vi "Zaber A Series Move.vi"() -> ()   [LabVIEW 2013]
doc: "This beginner example shows the Move VI, which allows the user to move devices based on real-world units easily."
uses:
  <instrlib>/Zaber A Series/Zaber A Series.lvlib
panel:
  in  "Units (0: microsteps)":u16(ring) items=["microsteps", "microns", "millimeters", "inches"]
  in  "Movement Type (0: relative)":u16(ring) items=["relative", "absolute"]
  in  "Device and Axis":string="1"
  in  "Microstep Size (0)":dbl=0.124023
  in  "Move Distance (0)":dbl
  in  "VISA resource name":refnum<visa-resource-name>="COM5"
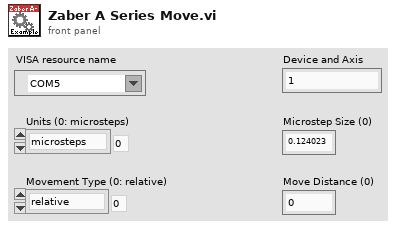
[diagram p1: front panel]
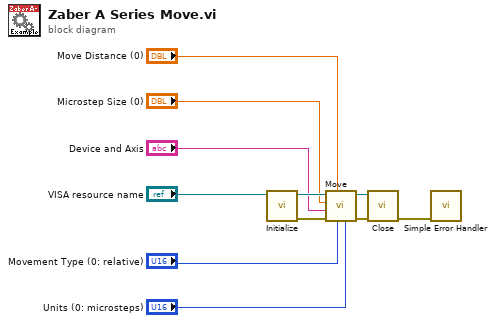
[diagram p0: block diagram]
diagram:
  n1 = call <instrlib>:"Initialize.vi"("VISA resource name"="VISA resource name") -> ("error out"=w8:errorcluster, "VISA resource name out"=w10:refnum<visa-resource-name>)  [unwired: 9 in]
  n2 = call <instrlib>:"Move.vi"("Units (0: microsteps)"="Units (0: microsteps)", "Movement Type (0: relative)"="Movement Type (0: relative)", "Move Distance (0)"="Move Distance (0)", "error in (no error)"=w8, "Device and Axis"="Device and Axis", "Microstep Size (0)"="Microstep Size (0)", "VISA resource name"=w10) -> ("error out"=w7:errorcluster, "VISA resource name out"=w9:refnum<visa-resource-name>)  [unwired: 3 in]
  n3 = call <instrlib>:"Close.vi"("error in (no error)"=w7, "VISA resource name"=w9) -> ("error out"=w6:errorcluster)  [unwired: 9 in]
  n4 = call <vilib>:"Simple Error Handler.vi"("error in (no error)"=w6) -> ()  [unwired: 4 in, 5 out]
